vi "Binary to Decimal.vi"(8 "error in":errorcluster, 11 "Binary Number ( 0 or 1)":i64 format="%b") -> (0 "error out":errorcluster, 3 "Decimal Number":i32)   [LabVIEW 2020]
doc: "This VI will convert Binary Values to Decimal Values."
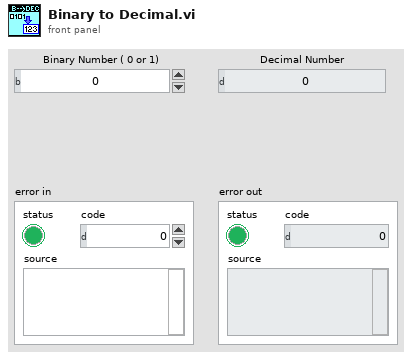
[diagram p1: front panel]
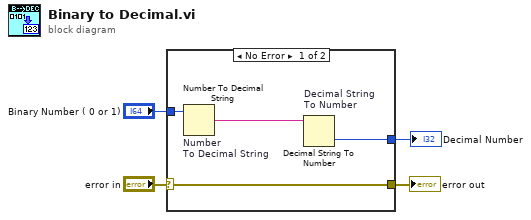
[diagram p0: block diagram]
diagram:
  n1 = case shown="No Error" "error in" {
    selector: "error in" -> [w8 w9]
    tunnel: "Binary Number ( 0 or 1)" -> [w7 _]
    tunnel: [w8 w9] -> w2
    tunnel: [w5 _] -> w1
    frame No Error {
      n2 = Number To Decimal String "Number \nTo Decimal String"(number=w7) -> (decimal integer string=w6:string)  [unwired: 1 in]
      n3 = Decimal String To Number "Decimal String \nTo Number"(string=w6) -> (number=w5:i32)  [unwired: 2 in, 1 out]
    }
    frame Error {
    }
  }
  "Decimal Number" <- w1
  "error out" <- w2
